vi "Configure.vi"(8 "error in (no error)":errorcluster, 9 "Record":bool, 10 "Recording Channels":refnum<k21>="All4498", 11 "AcquireTraces in":refnum<class "AcquireTraces.lvclass">) -> (0 "error out":errorcluster, 3 "AcquireTraces out":refnum<class "AcquireTraces.lvclass">)   [LabVIEW 2012, in "AcquireTraces.lvclass"]
uses:
  AcquireTraces.lvclass
  AcquireTraces.lvclass/AcquireTraces.ctl
  <vilib>/DAQmx/configure/timing.llb/DAQmx Timing (Sample Clock).vi
  <resource>/objmgr/daqmx.rc
panel:
  out "Name":refnum<k21>
  out "error out 2":errorcluster
  out "x/y":dbl
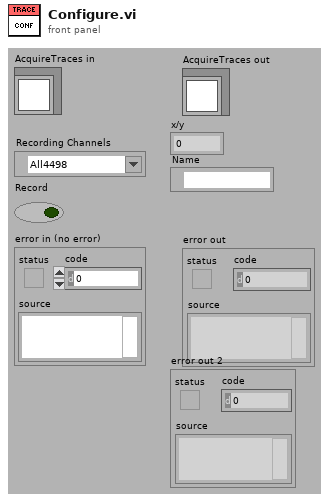
[diagram p1: front panel]
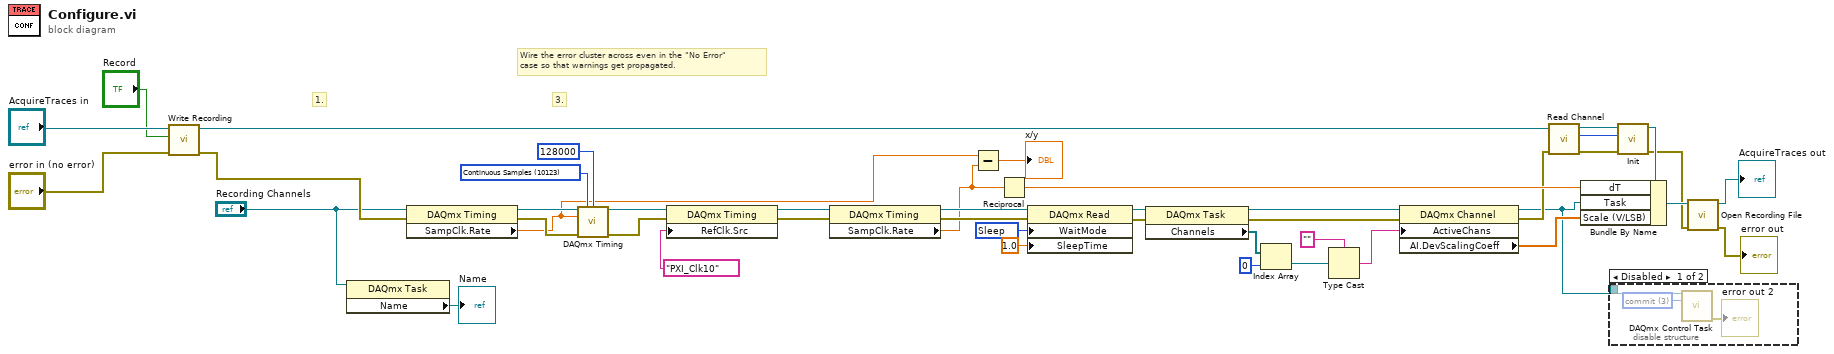
[diagram p0: block diagram]
diagram:
  w34 = 12547 items=["Wait For Interrupt"=12523, "Poll"=12524, "Yield"=12525, "Sleep"=12547] ("WaitMode")
  w38 = 10123 items=["Finite Samples"=10178, "Continuous Samples"=10123, "Hardware Timed Single Point"=12522] ("sample mode")
  # "3."
  # "1."
  # "Wire the error cluster across even in the \"No Error\"\ncase so that warnings get propagated."
  n1 = call-dynamic "Write Recording.vi"("error in (no error)"="error in (no error)", "Recording"="Record", "AcquireTraces in"="AcquireTraces in") -> ("error out"=w7:errorcluster, "AcquireTraces out"=w4:refnum<class "AcquireTraces.lvclass">)  [unwired: 7 in]
  n2 = property class="DAQmx Task"(reference="Recording Channels") -> ("Name"=→"Name":refnum<k21>)  [unwired: 1 in, 2 out]
  n3 = property class="DAQmx Timing"(reference="Recording Channels", error in=w7) -> (reference out=w21:refnum<k21>, error out=w22:errorcluster, "SampClk.Rate"=w14:dbl)
  n4 = call-poly <vilib>:"DAQmx Timing.vi"("task/channels in"=w21, "sample mode"=w38, "samples per channel"=128000, "rate"=w14, "error in"=w22) -> ("task out"=w12:refnum<k21>, "error out"=w10:errorcluster)  [unwired: 9 in]
  n5 = property class="DAQmx Timing"(reference=w12, error in=w10, "RefClk.Src"=tag "PXI_Clk10") -> (reference out=w11:refnum<k21>, error out=w9:errorcluster)
  n6 = property class="DAQmx Timing"(reference=w11, error in=w9) -> (reference out=w36:refnum<k21>, error out=w33:errorcluster, "SampClk.Rate"=w15:dbl)
  n7 = Subtract(x=w14, y=w15) -> (x-y=→"x/y":dbl)
  n8 = Reciprocal(x=w15) -> (1/x=w32:dbl)
  n9 = property class="DAQmx Read"(reference=w36, error in=w33, "WaitMode"=w34, "SleepTime"=1.0) -> (reference out=w30:refnum<k21>, error out=w29:errorcluster)
  n10 = property class="DAQmx Task"(reference=w30, error in=w29) -> (reference out=w28:refnum<k21>, error out=w27:errorcluster, "Channels"=w20:refnum<k21>[])
  n11 = Index Array(array=w20, index=0) -> (element=w25:refnum<k21>)
  n12 = Type Cast(type="", x=w25) -> (*(type *) &x=w23:string)
  n13 = property class="DAQmx Channel"(reference=w28, error in=w27, "ActiveChans"=w23) -> (reference out=w3:refnum<k21>, error out=w6:errorcluster, "AI.DevScalingCoeff"=w19:dbl[])
  n14 = call-dynamic "Read Channel.vi"("error in (no error)"=w6, "AcquistionObject in"=w4) -> ("error out"=w39:errorcluster, "Channel"=w41:i16, "AcquistionObject out"=w40:refnum<class "AcquireTraces.lvclass">)  [unwired: 7 in]
  n15 = disable-structure shown="Disabled" {
    disable-tunnel: w3 -> [w47 _]
    frame Disabled {
      w46 = 3 items=["verify"=2, "reserve"=4, "commit"=3, "unreserve"=5, "abort"=6] ("action")
      n16 = call <vilib>:"DAQmx Control Task.vi"("task/channels in"=w47, "action"=w46) -> ("error out"=→"error out 2":errorcluster)  [unwired: 12 in, 1 out]
    }
    frame Enabled {
    }
  }
  n17 = call-dynamic "Init.vi"("error in (no error)"=w39, "Channel"=w41, "AcquistionObject in"=w40) -> ("error out"=w5:errorcluster, "AcquistionObject out"=w44:refnum<class "AcquireTraces.lvclass">)  [unwired: 7 in]
  n18 = Bundle By Name(cluster=w44, "dT"=w32, "Task"=w3, "Scale (V/LSB)"=w19) -> (w31:refnum<class "AcquireTraces.lvclass">)
  n19 = call "Open Recording File.vi"("error in (no error)"=w5, "AcquireTraces In"=w31) -> ("error out"=→"error out":errorcluster, "AcquireTraces Out"=→"AcquireTraces out":refnum<class "AcquireTraces.lvclass">)  [unwired: 8 in]
